vi "RSZVB Get Pulse Section Limit Lines State.vi"(5 "Record Number (1)":i32=1, 6 "Generator/Port Number (1)":i32=1, 7 "Interface Type (0: Generator)":i32(ring) items=["Generator", "Analyzer Source"], 8 "error in (no error)":errorcluster {"code" format="%.0x"}, 9 "Receiver Type (0: A)":i32(ring) items=["A", "B"], 10 "Channel (1)":i32=1, 11 "VISA session":refnum<visa-resource-name>) -> (0 "error out":errorcluster {"code" format="%.0x"}, 1 "Limit Lines State":bool, 3 "dup VISA session":refnum<visa-resource-name>)   [LabVIEW 2011]
doc: "This VI returns the limit lines state of the averaging section for the wave quantity. \n\nRemote-control command(s):\n[SENSe<Ch>:]PULSe:RECeiver:A<rec_no>:GENerator<gen_no>:LINEs[:STATe]?\n[SENSe<Ch>:]PULSe:RECeiver:A<rec_no>:SRCPort<port_no>:LINEs[:STATe]?\n[SENSe<Ch>:]PULSe:RECeiver:B<rec_no>:GENerator<gen_no>:LINEs[:STATe]?\n[SENSe<Ch>:]PULSe:RECeiver:B<rec_no>:SRCPort<port_no>:LINEs[:STATe]?"
uses:
  _utility/RSZVB Global Data.vi
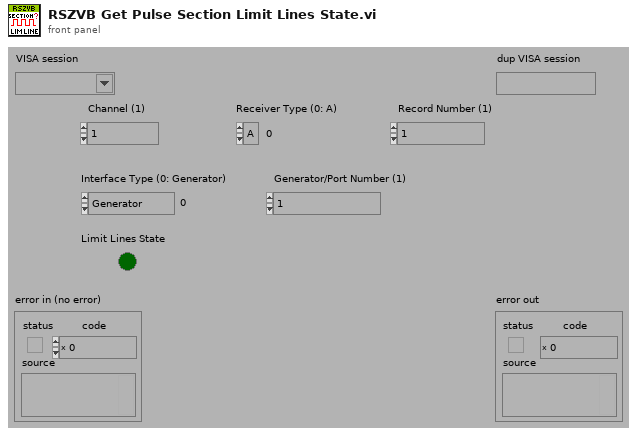
[diagram p1: front panel]
types:
  T1 = cluster{"Error Checking (T: On)":bool, "Installed Options":string[], "Data Valid?":bool, "Ports":i32, "Model":string[], "Option Checking (T: On)":bool}[]
  T2 = cluster{"Error Checking (T: On)":bool, "Installed Options":string[], "Data Valid?":bool, "Ports":i32, "Model":string[], "Option Checking (T: On)":bool}
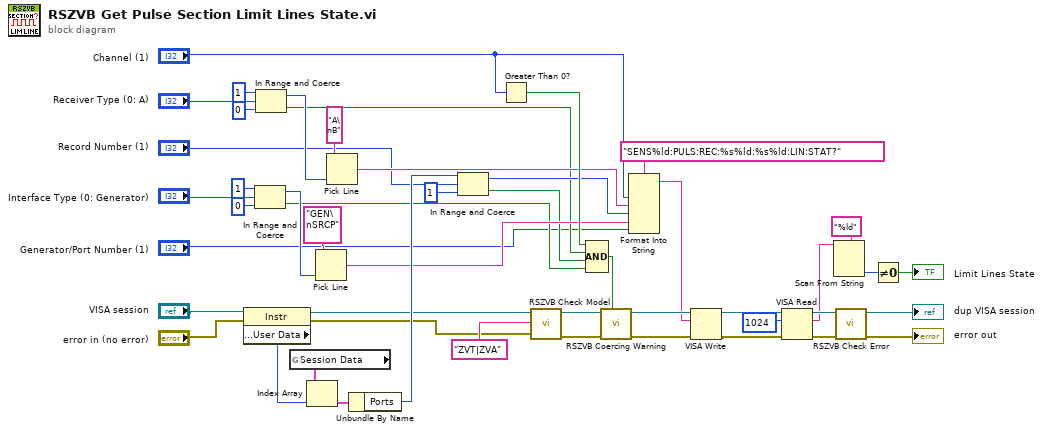
[diagram p0: block diagram]
diagram:
  n1 = property class="Instr"(reference="VISA session", error in="error in (no error)") -> (reference out=w27:refnum<visa-resource-name>, error out=w26:errorcluster, "General Settings:User Data"=w29:u32)
  n2 = In Range and Coerce(upper limit=1, x="Interface Type (0: Generator)", lower limit=0) -> (coerced(x)=w32:i32, In Range?=w19:bool)
  n3 = In Range and Coerce(upper limit=1, x="Receiver Type (0: A)", lower limit=0) -> (coerced(x)=w36:i32, In Range?=w21:bool)
  n4 = global read "RSZVB Global Data.vi" "Session Data"() -> (w30:T1)
  n5 = Index Array(array=w30, index=w29) -> (element=w31:T2)
  n6 = Pick Line(multi-line string="GEN\nSRCP", line index=w32) -> (output string=w22:string)  [unwired: 1 in]
  n7 = Pick Line(multi-line string="A\nB", line index=w36) -> (output string=w24:string)  [unwired: 1 in]
  n8 = Unbundle By Name(w31) -> ("Ports"=w28:i32)
  n9 = In Range and Coerce(upper limit=w28, x="Record Number (1)", lower limit=1) -> (coerced(x)=w23:i32, In Range?=w20:bool)
  n10 = Greater Than 0?(x="Channel (1)") -> (x > 0?=w43:bool)
  n11 = call "RSZVB Check Model.vi"("error in (no error)"=w26, "Model"="ZVT|ZVA" ("Options"), "VISA session"=w27) -> ("error out"=w41:errorcluster, "dup VISA session"=w40:refnum<visa-resource-name>)  [unwired: 7 in]
  n12 = Compound Arithmetic op=AND(w43, w21, w20, w19) -> (w45:bool)
  n13 = call "RSZVB Coercing Warning.vi"("In Range?"=w45, "error in (no error)"=w41, "VISA session"=w40) -> ("error out"=w46:errorcluster, "dup VISA session"=w47:refnum<visa-resource-name>)  [unwired: 7 in]
  n14 = Format Into String(format string="SENS%ld:PULS:REC:%s%ld:%s%ld:LIN:STAT?", "Channel (1)", w24, w23, w22, "Generator/Port Number (1)") -> (resulting string=w44:string)  [unwired: 2 in, 1 out]
  n15 = VISA Write(VISA resource name=w47, write buffer=w44, error in (no error)=w46) -> (VISA resource name out=w4:refnum<visa-resource-name>, error out=w5:errorcluster)  [unwired: 1 out]
  n16 = VISA Read(VISA resource name=w4, byte count=u32 1024 ("byte count (0)"), error in (no error)=w5) -> (VISA resource name out=w10:refnum<visa-resource-name>, read buffer=w7:string, error out=w9:errorcluster)  [unwired: 1 out]
  n17 = Scan From String(format string="%ld", input string=w7) -> (output 1=w6:i32)  [unwired: 3 in, 3 out]
  n18 = call "RSZVB Check Error.vi"("error in (no error)"=w9, "VISA session"=w10) -> ("error out"=→"error out":errorcluster, "dup VISA session"=→"dup VISA session":refnum<visa-resource-name>)  [unwired: 8 in]
  n19 = Not Equal To 0?(x=w6) -> (x != 0?=→"Limit Lines State":bool)
